vi "Test Zental PC  from Config file.vi"() -> ()   [LabVIEW 2009]
uses:
  LV-BME Interface/ChnlSettings.ctl
  DG Classes/BME_DG_Base/BME_DG_Base.lvclass
  DG Classes/BME_DG_Chnl/BME_DG_Chnl.lvclass
  DG Classes/BME_DG_System/BME_DG_System.lvclass
  POLARIS BME DG.lvlib
panel:
  out "error out 2":errorcluster
  in  "pathCalFiles":path=path "C:/CS Framework/LVSCC/LV2009/GPL/Projects/cs-framework/CSClass/CSPOLARIS/POLARIS BME DG"
  in  "pathParameterFile":path=path "C:/CS Framework/LVSCC/LV2009/GPL/Projects/cs-framework/CSClass/CSPOLARIS/POLARIS BME DG/test config  file.xml"
  out "stop error":errorcluster
  out "Problem Chnls out":string[](array[string])
  out "DelayFormulas":string[](array[string])=[" 10000.0095", "Delay Offset +0.819", "Pulspicker On + 0.013"]
  in  "Reset Error":bool
  out "error out":errorcluster
  in  "Update Delay formula":bool=TRUE
  in  "DelayFormula":string=" 10000.0095"
  in  "Aknowledge interrupts":bool=TRUE
  in  "stop 3":bool=TRUE
  in  "SetDelay":bool=TRUE
  in  "UpdateChnl":bool=TRUE
  in  "ChnlParameter":T2 {"ChnParam2write"."Delay (µs)" min=0.0 max=100000000.0 format="%.5f"}
  out "CountsRemains":i32=2147483647
  out "TriggerCounters":i32[](array[numeric])=[281, 0, 0, 0, -533591008, 0, 0, 0, 0]
  out "Interrupts":u32[](array[numeric])=[11153, 10240, 10240, 10240, 11008, 11008, 10240, 10240, 10240] format="%b"
  out "RemainingTriggers":T3(array[cluster])=[[{"Time Stamp"=timestamp(3421911180.6875 s since 1904-01-01), "Numeric"=1}, {"Time Stamp"=timestamp(3421911180.6875 s since 1904-01-01), "Numeric"=1}, {"Time Stamp"=timestamp(3421911180.6875 s since 1904-01-01), "Numeric"=1}, {"Time Stamp"=timestamp(3421911180.6875 s since 1904-01-01), "Numeric"=1}, {"Time Stamp"=timestamp(3421911180.6875 s since 1904-01-01), "Numeric"=9}, {"Time Stamp"=timestamp(3421911180.6875 s since 1904-01-01), "Numeric"=1}, {"Time Stamp"=timestamp(3421911180.6875 s since 1904-01-01), "Numeric"=1}, {"Time Stamp"=timestamp(3421911180.6875 s since 1904-01-01), "Numeric"=1}, {"Time Stamp"=timestamp(3421911180.6875 s since 1904-01-01), "Numeric"=1}], [{"Time Stamp"=timestamp(3421911180.6875 s since 1904-01-01), "Numeric"=10}, {"Time Stamp"=timestamp(3421911180.6875 s since 1904-01-01), "Numeric"=1}, {"Time Stamp"=timestamp(3421911180.6875 s since 1904-01-01), "Numeric"=1}, {"Time Stamp"=timestamp(3421911180.6875 s since 1904-01-01), "Numeric"=1}, {"Time Stamp"=timestamp(3421911180.6875 s since 1904-01-01), "Numeric"=9}, {"Time Stamp"=timestamp(3421911180.6875 s since 1904-01-01), "Numeric"=1}, {"Time Stamp"=timestamp(3421911180.6875 s since 1904-01-01), "Numeric"=1}, {"Time Stamp"=timestamp(3421911180.6875 s since 1904-01-01), "Numeric"=1}, {"Time Stamp"=timestamp(3421911180.6875 s since 1904-01-01), "Numeric"=1}], [{"Time Stamp"=timestamp(3421911180.6875 s since 1904-01-01), "Numeric"=10}, {"Time Stamp"=timestamp(3421911180.6875 s since 1904-01-01), "Numeric"=1}, {"Time Stamp"=timestamp(3421911180.6875 s since 1904-01-01), "Numeric"=1}, {"Time Stamp"=timestamp(3421911180.6875 s since 1904-01-01), "Numeric"=1}, {"Time Stamp"=timestamp(3421911180.6875 s since 1904-01-01), "Numeric"=609}, {"Time Stamp"=timestamp(3421911180.6875 s since 1904-01-01), "Numeric"=1}, {"Time Stamp"=timestamp(3421911180.6875 s since 1904-01-01), "Numeric"=1}, {"Time Stamp"=timestamp(3421911180.6875 s since 1904-01-01), "Numeric"=1}, {"Time Stamp"=timestamp(3421911180.6875 s since 1904-01-01), "Numeric"=1}]] {"Time Stamp" format="%<%I:%M:%S%3u %p>T"}
  in  "stop 2":bool=TRUE
  in  "ReadStatus":bool=TRUE
  in  "Activate":bool=TRUE
  in  "ResetModuloCounters":bool=TRUE
  in  "TriggerModulo":u32=4
  out "Modulo Settings":u32[](array[numeric])=[1, 10, 10]
  out "Chnls":T1[](array[typedef])=[{" Delay (µs)"=10000.0095, "On?"=TRUE, "PositiveVoltage?"=TRUE, "50OhmTerminated? "=TRUE, "25OhmOutput?"=FALSE}, {" Delay (µs)"=10000.829, "On?"=TRUE, "PositiveVoltage?"=TRUE, "50OhmTerminated? "=TRUE, "25OhmOutput?"=FALSE}, {" Delay (µs)"=10000.843, "On?"=TRUE, "PositiveVoltage?"=TRUE, "50OhmTerminated? "=TRUE, "25OhmOutput?"=FALSE}] {"Delay (µs)" min=0.0 max=100000000.0 format="%.5f"}
  in  "Selected Chnl":u16(ring)
  in  "Selected Card":u16(ring) items=["Master", "Servant"]
  in  "STOP":bool
  in  "ChnParam2write":T1={" Delay (µs)"=0.0, "On?"=TRUE, "PositiveVoltage?"=TRUE, "50OhmTerminated? "=TRUE, "25OhmOutput?"=FALSE} {"Delay (µs)" min=0.0 max=100000000.0 format="%.5f"}
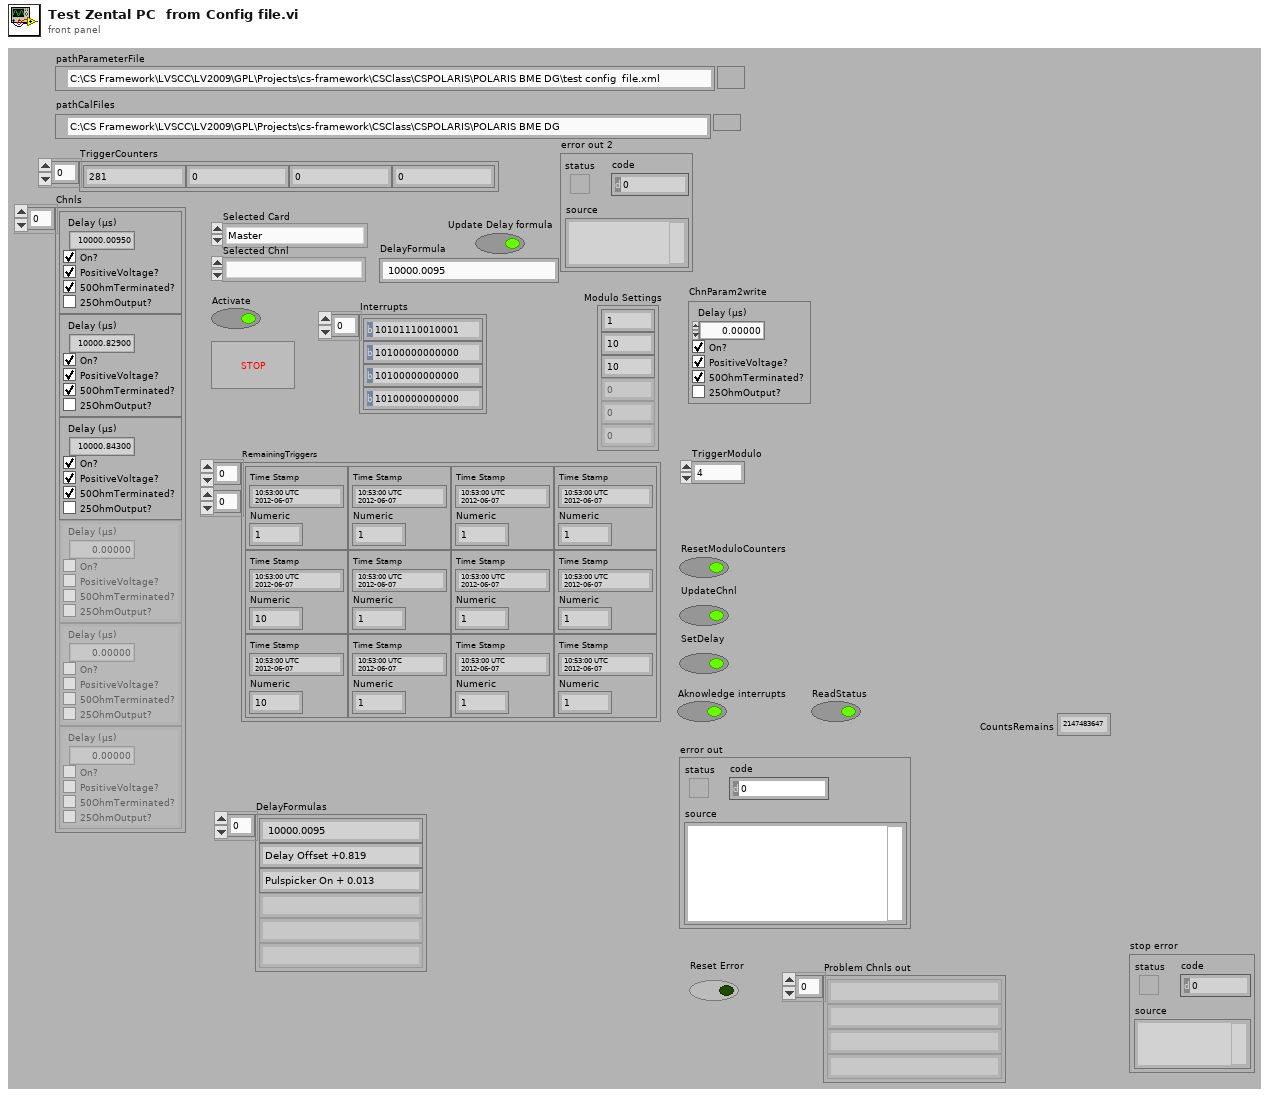
[diagram p1: front panel]
types:
  T1 = typedef "POLARIS BME DG.lvlib/ChnlSettings.ctl" = cluster{" Delay (µs)":dbl, "On?":bool, "PositiveVoltage?":bool, "50OhmTerminated? ":bool, "25OhmOutput?":bool}
  T2 = cluster{"ChnlName":string, "ChnParam2write":T1, "TriggerModulo":u32}
  T3 = cluster{"Time Stamp":timestamp, "Numeric":i32}[][]
  T4 = enum8{"Enabled", "Disabled", "Disabled and Grayed Out"}
  T5 = typedef "POLARIS BME DG.lvlib/BME_DG_TriggerSettings.ctl" = cluster{"Clock Source":T6, " clock modulo":u32, "TriggerEnabled?":bool, "trigger modulo ":i32, "InputTerminated?":bool, "Inhibit(µs)":dbl, "TriggerLevel":dbl, "PresetValue":i32, "InternalTrigger?":bool, "InternalArm?":bool, "SWTrigger?":bool, "RisingEdge?":bool, "StopOnPreset?":bool, "ResetWhenDone?":bool, "Gate Divider":i32, "PositiveGate?":bool}
  T6 = typedef "POLARIS BME DG.lvlib/ClockSource.ctl" = i32
  T7 = cluster{"ChnlName":string, "ChnParam2write":T1, "TriggerModulo":u32}[]
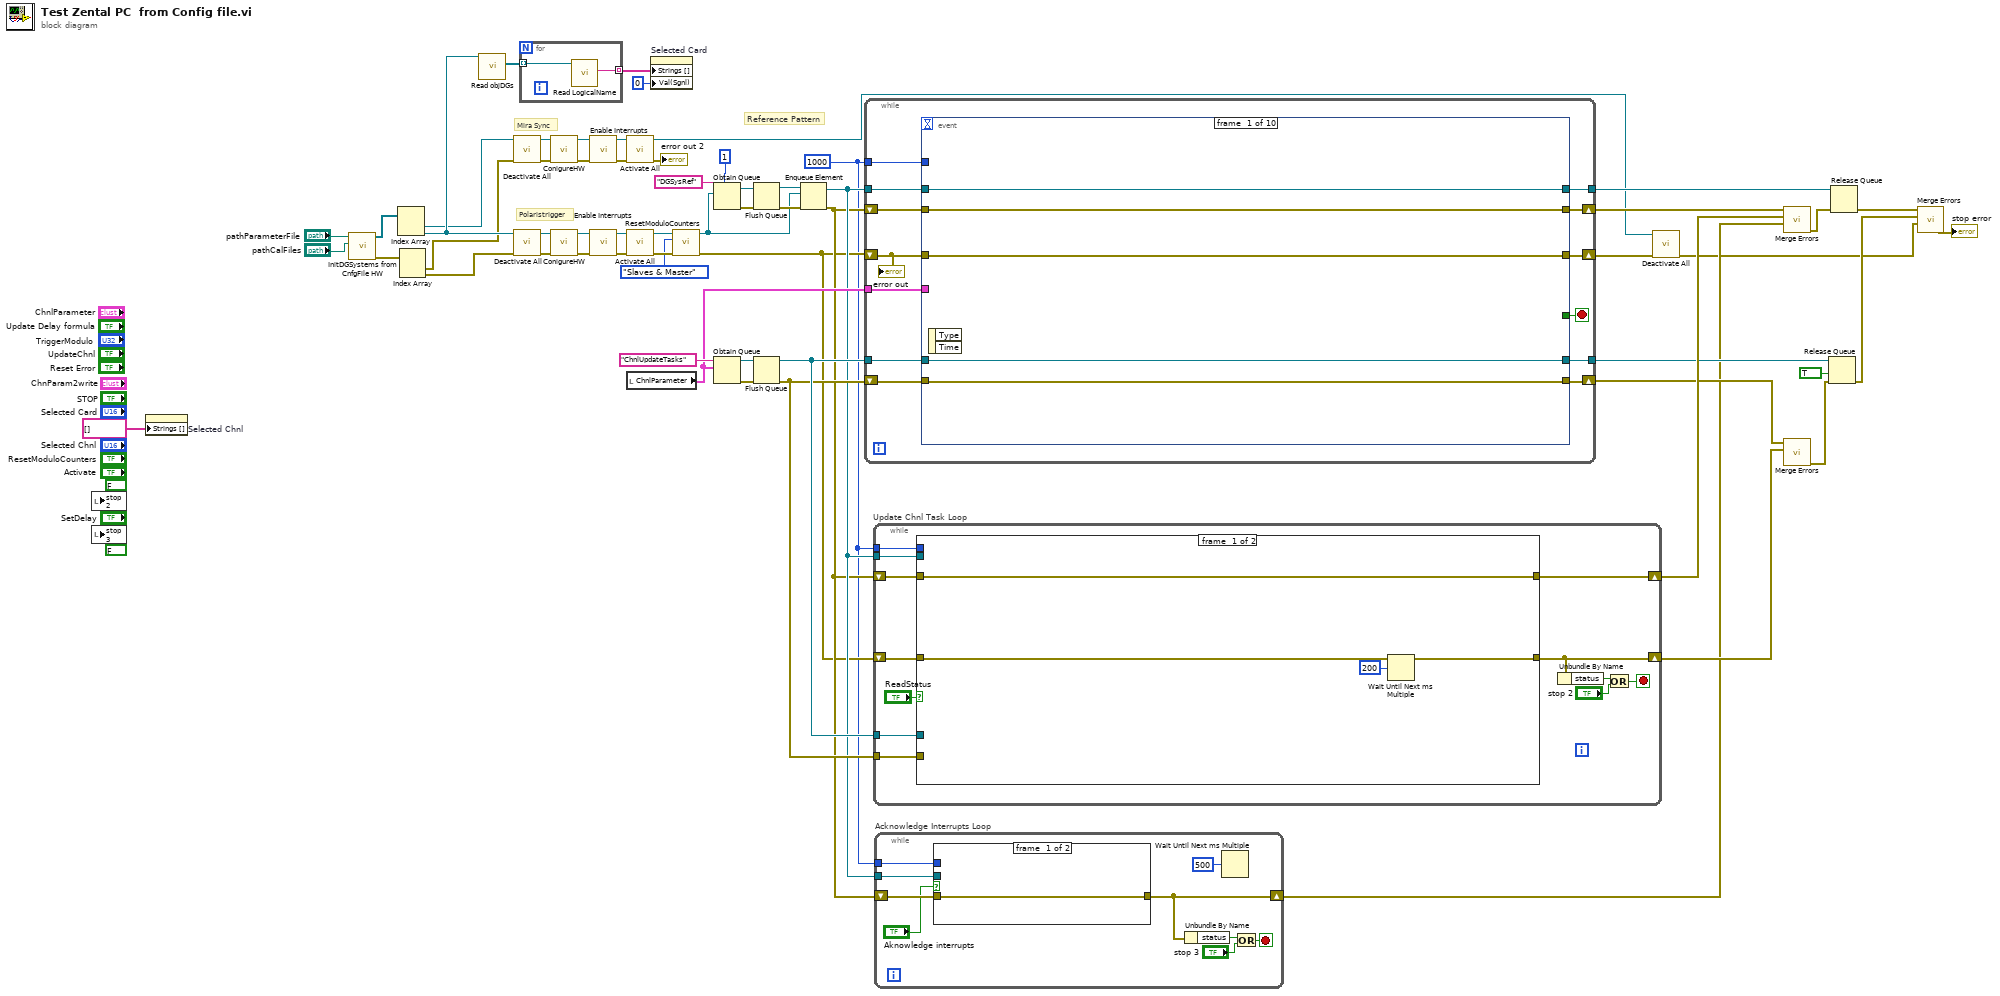
[diagram p0: block diagram]
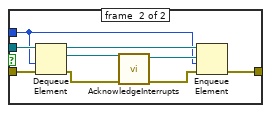
[diagram p2: hidden frame]
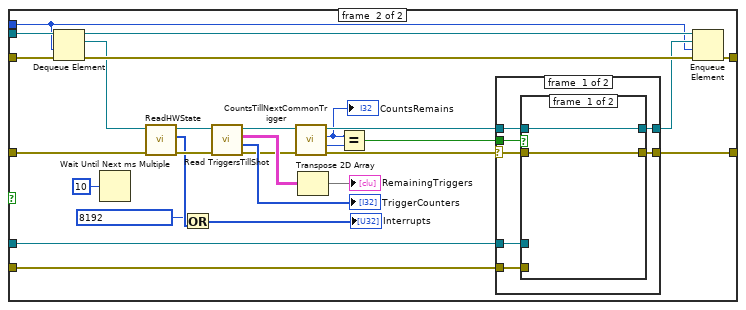
[diagram p3: hidden frame]
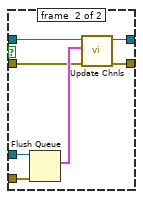
[diagram p4: hidden frame]
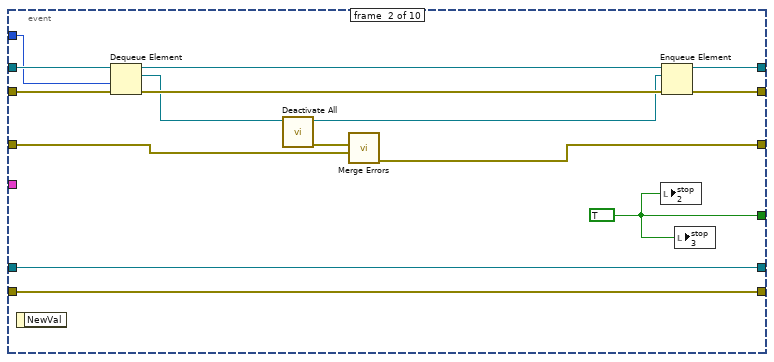
[diagram p6: hidden frame]
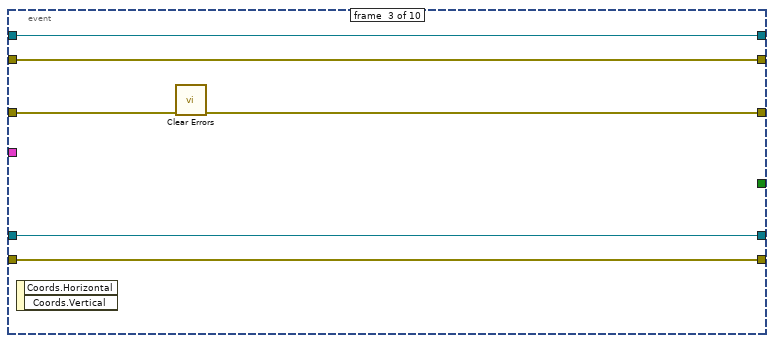
[diagram p7: hidden frame]
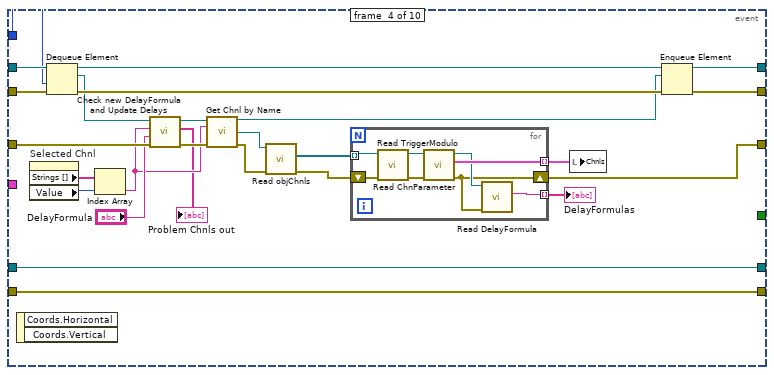
[diagram p8: hidden frame]
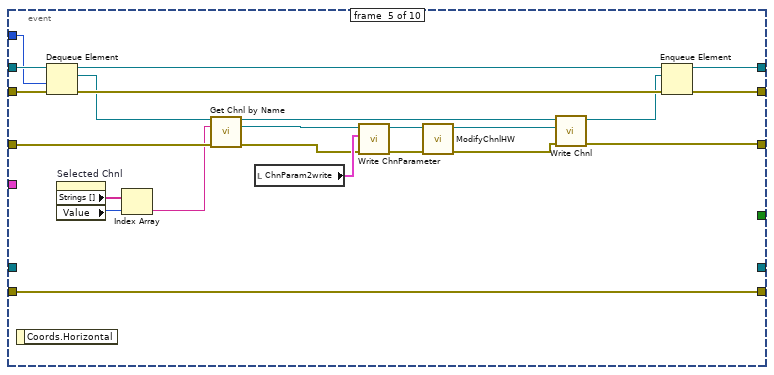
[diagram p9: hidden frame]
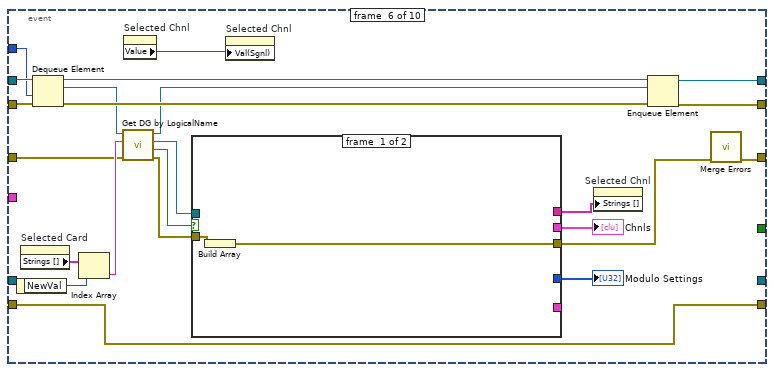
[diagram p10: hidden frame]
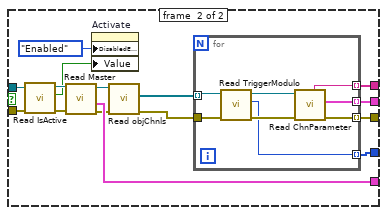
[diagram p11: hidden frame]
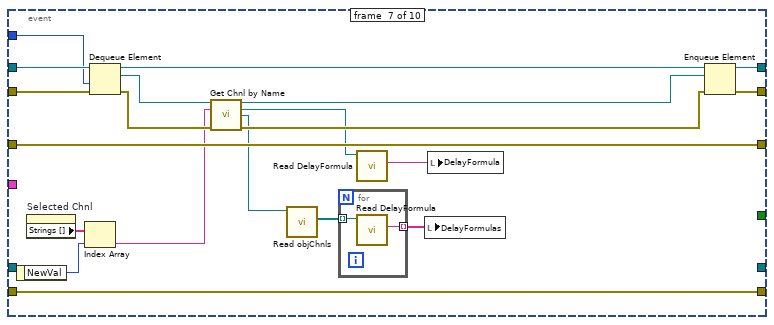
[diagram p12: hidden frame]
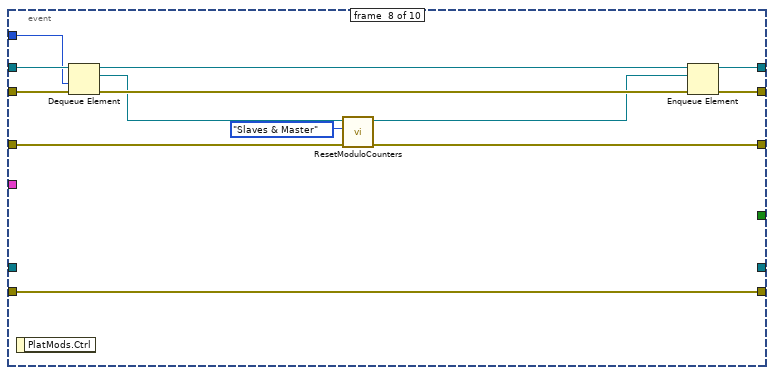
[diagram p13: hidden frame]
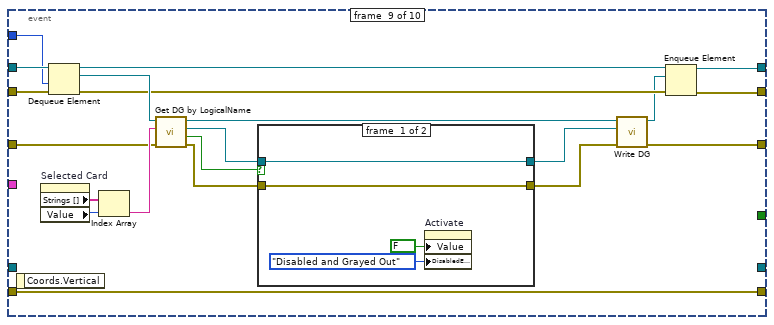
[diagram p14: hidden frame]
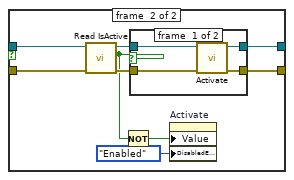
[diagram p15: hidden frame]
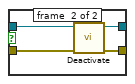
[diagram p16: hidden frame]
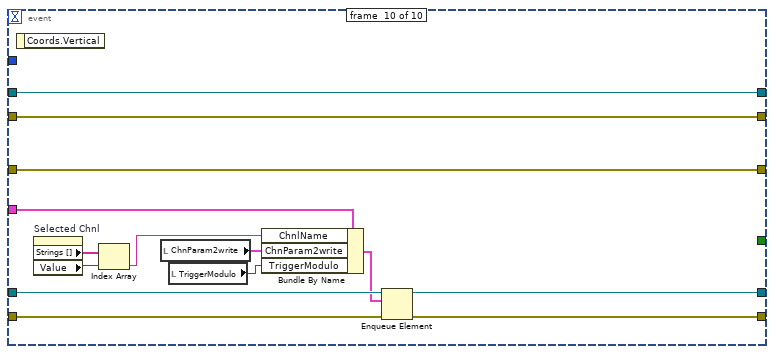
[diagram p17: hidden frame]
diagram:
  w21 = 1000 ("timeout in ms (-1)")
  # "Polaristrigger"
  # "Mira Sync"
  # "Reference Pattern"
  n1 = local write "stop 2"(FALSE ("stop 2")) -> ()
  n2 = local write "stop 3"(FALSE ("stop 3")) -> ()
  n3 = property on="Selected Chnl" class="Ring (strict)"("Strings []"=string[] []) -> ()  [unwired: 2 in, 2 out]
  n4 = call "InitDGSystems from CnfgFile HW.vi"("pathCalibrConsts"="pathCalFiles", "Config File"="pathParameterFile") -> ("Errors"=w7:errorcluster[], "DG Systems"=w16:refnum<class "BME_DG_System.lvclass">[])  [unwired: 8 in]
  n5 = Index Array(array=w16) -> (element #1=w8:refnum<class "BME_DG_System.lvclass">, element #2=w15:refnum<class "BME_DG_System.lvclass">)  [unwired: 2 in]
  n6 = Index Array(array=w7) -> (element #1=w5:errorcluster, element #2=w6:errorcluster)  [unwired: 2 in]
  n7 = call "Read objDGs.vi"("BME_DG_System in"=w15) -> ("objDGs"=w20:refnum<class "BME_DG_Base.lvclass">[])  [unwired: 8 in, 2 out]
  n8 = call "Deactivate All.vi"("error in (no error)"=w5, "BME_DG_System in"=w8) -> ("error out"=w10:errorcluster, "BME_DG_System out"=w9:refnum<class "BME_DG_System.lvclass">)  [unwired: 8 in]
  n9 = call "Deactivate All.vi"("error in (no error)"=w6, "BME_DG_System in"=w15) -> ("error out"=w38:errorcluster, "BME_DG_System out"=w39:refnum<class "BME_DG_System.lvclass">)  [unwired: 8 in]
  n10 = for {
    tunnel: w20 -> [w65] mode=indexing
    tunnel: [w64] -> w19 mode=indexing
    n11 = call "Read LogicalName.vi"("BME_DG_Base in"=w65) -> ("LogicalName"=w64:string)  [unwired: 8 in, 2 out]
  }
  n12 = call "ConigureHW.vi"("error in (no error)"=w10, "BME_DG_System in"=w9) -> ("error out"=w12:errorcluster, "BME_DG_System out"=w11:refnum<class "BME_DG_System.lvclass">)  [unwired: 8 in]
  n13 = call "ConigureHW.vi"("error in (no error)"=w38, "BME_DG_System in"=w39) -> ("error out"=w36:errorcluster, "BME_DG_System out"=w37:refnum<class "BME_DG_System.lvclass">)  [unwired: 8 in]
  n14 = call "Enable Interrupts.vi"("error in (no error)"=w12, "BME_DG_System in"=w11) -> ("error out"=w14:errorcluster, "BME_DG_System out"=w13:refnum<class "BME_DG_System.lvclass">)  [unwired: 8 in]
  n15 = call "Enable Interrupts.vi"("error in (no error)"=w36, "BME_DG_System in"=w37) -> ("error out"=w30:errorcluster, "BME_DG_System out"=w31:refnum<class "BME_DG_System.lvclass">)  [unwired: 8 in]
  n16 = call "Activate All.vi"("error in (no error)"=w14, "BME_DG_System in"=w13) -> ("error out"=→"error out 2":errorcluster, "BME_DG_System out"=w2:refnum<class "BME_DG_System.lvclass">)  [unwired: 8 in]
  n17 = call "Activate All.vi"("error in (no error)"=w30, "BME_DG_System in"=w31) -> ("error out"=w27:errorcluster, "BME_DG_System out"=w29:refnum<class "BME_DG_System.lvclass">)  [unwired: 8 in]
  n18 = local read "ChnlParameter"() -> (w47:T2)
  n19 = property on="Selected Card" class="Ring (strict)"("Strings []"=w19, "Val(Sgnl)"=u16 0 ("Value (Signaling)")) -> ()  [unwired: 2 in, 2 out]
  n20 = call "ResetModuloCounters.vi"("error in (no error)"=w27, "Enum"=enum16{"Slaves only", "Slaves & Master"}."Slaves & Master", "BME_DG_System in"=w29) -> ("error out"=w26:errorcluster, "BME_DG_System out"=w28:refnum<class "BME_DG_System.lvclass">)  [unwired: 7 in]
  n21 = Obtain Queue(max queue size (-1, unlimited)=1, name (unnamed)="DGSysRef", element data type=w28) -> (queue out=w55:refnum<queue>, error out=w53:errorcluster)  [unwired: 2 in, 1 out]
  n22 = Obtain Queue(name (unnamed)="ChnlUpdateTasks", element data type=w47) -> (queue out=w48:refnum<queue>, error out=w49:errorcluster)  [unwired: 3 in, 1 out]
  n23 = Flush Queue(queue=w55, error in (no error)=w53) -> (queue out=w54:refnum<queue>, error out=w52:errorcluster)  [unwired: 1 out]
  n24 = Flush Queue(queue=w48, error in (no error)=w49) -> (queue out=w44:refnum<queue>, error out=w43:errorcluster)  [unwired: 1 out]
  n25 = Enqueue Element(queue=w54, element=w28, error in (no error)=w52) -> (queue out=w35:refnum<queue>, error out=w34:errorcluster)  [unwired: 1 in, 1 out]
  n26 = while {
    shift-right: [w74] -> w4
    shift-left: w26 -> [w76]
    shift-right: [w72] -> w58
    shift-left: w34 -> [w73]
    tunnel: w35 -> [w77]
    tunnel: [w75] -> w60
    tunnel: w44 -> [w71]
    tunnel: w47 -> [w70]
    tunnel: [w68] -> w46
    shift-right: [w67] -> w42
    shift-left: w43 -> [w69]
    tunnel: w21 -> [w66]
    stop <- w78 stop-if-true
    n27 = event shown="[5] \"Selected Card\": Value Change" {
      selector: _ -> [_ _ _ _ _ _ _ _ _ _]
      dyn-events: _ -> [_ _ _ _ _ _ _ _ _ _]
      timeout: _ -> [_ _ _ _ _ _ _ _ _ _]
      tunnel: [_ w87 _ _ _ _ _ _ _ _] -> w78
      tunnel: w77 -> [w83 w96 w103 w129 w160 w173 w224 w244 w254 w300]
      tunnel: w76 -> [w82 w85 w104 w121 w151 w181 w229 w234 w262 w299]
      tunnel: [w83 w92 w103 w125 w156 w171 w222 w239 w248 w300] -> w75
      tunnel: [w82 w86 w99 w109 w140 w166 w229 w235 w255 w299] -> w74
      tunnel: w73 -> [w81 w95 w102 w128 w159 w172 w223 w242 w253 w296]
      tunnel: [w81 w93 w102 w126 w157 w170 w221 w240 w247 w296] -> w72
      tunnel: w71 -> [w80 w89 w101 w124 _ _ _ _ _ w291]
      tunnel: w70 -> [_ _ _ _ _ _ _ _ _ w295]
      tunnel: w69 -> [w79 w88 w100 w123 w155 w164 w228 w238 w246 w289]
      tunnel: [w80 w89 w101 w124 _ _ _ _ _ w288] -> w68
      tunnel: [w79 w88 w100 w123 w155 w164 w228 w238 w246 w287] -> w67
      tunnel: w66 -> [_ w84 _ w105 w139 w162 w210 w232 w245 _]
      event #0 {
        n28 = event-data() -> ()  [unwired: 1 in, 2 out]
      }
      event #1 {
        w87 = TRUE
        n29 = event-data() -> ()  [unwired: 1 in, 1 out]
        n30 = Dequeue Element(queue=w96, timeout in ms (-1)=w84, error in (no error)=w95) -> (queue out=w97:refnum<queue>, element=w90:refnum<class "BME_DG_System.lvclass">, error out=w94:errorcluster)  [unwired: 1 out]
        n31 = call "Deactivate All.vi"("BME_DG_System in"=w90) -> ("error out"=w98:errorcluster, "BME_DG_System out"=w91:refnum<class "BME_DG_System.lvclass">)  [unwired: 9 in]
        n32 = call <vilib>:"Merge Errors.vi"("error in 3 (no error)"=w85, "error in 2 (no error)"=w98) -> ("error out"=w86:errorcluster)  [unwired: 5 in]
        n33 = local write "stop 2"(w87) -> ()
        n34 = Enqueue Element(queue=w97, element=w91, error in (no error)=w94) -> (queue out=w92:refnum<queue>, error out=w93:errorcluster)  [unwired: 1 in, 1 out]
        n35 = local write "stop 3"(w87) -> ()
      }
      event #2 {
        n36 = event-data() -> ()  [unwired: 1 in, 2 out]
        n37 = call <vilib>:"Clear Errors.vi"("error in (no error)"=w104) -> ("error out"=w99:errorcluster)  [unwired: 6 in]
      }
      event #3 {
        n38 = event-data() -> ()  [unwired: 1 in, 2 out]
        n39 = property on="Selected Chnl" class="Ring (strict)"() -> ("Strings []"=w119:string[], "Value"=w120:u16)  [unwired: 2 in, 2 out]
        n40 = Dequeue Element(queue=w129, timeout in ms (-1)=w105, error in (no error)=w128) -> (queue out=w130:refnum<queue>, element=w122:refnum<class "BME_DG_System.lvclass">, error out=w127:errorcluster)  [unwired: 1 out]
        n41 = Index Array(array=w119, index=w120) -> (element=w108:string)
        n42 = call "Check new DelayFormula and Update Delays.vi"("error in (no error)"=w121, "Delay Formula"="DelayFormula", "ChnlName"=w108, "BME_DG_System in"=w122) -> ("error out"=w111:errorcluster, "Problem Chnls out"=→"Problem Chnls out":string[], "BME_DG_System out"=w113:refnum<class "BME_DG_System.lvclass">)  [unwired: 5 in]
        n43 = call "Get Chnl by Name.vi"("BME_DG_System in"=w113, "Chnl Name"=w108, "error in (no error)"=w111) -> ("BME_DG_System out"=w112:refnum<class "BME_DG_System.lvclass">, "Owner DG"=w114:refnum<class "BME_DG_Base.lvclass">, "error out"=w110:errorcluster)  [unwired: 7 in, 3 out]
        n44 = call-dynamic "Read objChnls.vi"("error in (no error)"=w110, "BME_DG_Base in"=w114) -> ("error out"=w115:errorcluster, "objChnls"=w117:refnum<class "BME_DG_Chnl.lvclass">[])  [unwired: 6 in, 2 out]
        n45 = for {
          tunnel: w117 -> [w137] mode=indexing
          tunnel: [w138] -> w116 mode=indexing
          shift-right: [w132] -> w109
          shift-left: w115 -> [w135]
          tunnel: [w131] -> w107 mode=indexing
          n46 = call-dynamic "Read TriggerModulo.vi"("error in (no error)"=w135, "BME_DG_Chnl in"=w137) -> ("error out"=w134:errorcluster, "BME_DG_Chnl out"=w136:refnum<class "BME_DG_Chnl.lvclass">)  [unwired: 7 in, 1 out]
          n47 = call-dynamic "Read ChnParameter.vi"("error in (no error)"=w134, "BME_DG_Chnl in"=w136) -> ("error out"=w132:errorcluster, "ChnParemater"=w138:T1, "BME_DG_Chnl out"=w133:refnum<class "BME_DG_Chnl.lvclass">)  [unwired: 4 in, 3 out]
          n48 = call-dynamic "Read DelayFormula.vi"("error in (no error)"=w132, "BME_DG_Chnl in"=w133) -> ("DelayFormula"=w131:string)  [unwired: 7 in, 2 out]
        }
        "DelayFormulas" <- w107
        n49 = local write "Chnls"(w116) -> ()
        n50 = Enqueue Element(queue=w130, element=w112, error in (no error)=w127) -> (queue out=w125:refnum<queue>, error out=w126:errorcluster)  [unwired: 1 in, 1 out]
      }
      event #4 {
        n51 = event-data() -> ()  [unwired: 1 in, 1 out]
        n52 = Dequeue Element(queue=w160, timeout in ms (-1)=w139, error in (no error)=w159) -> (queue out=w161:refnum<queue>, element=w152:refnum<class "BME_DG_System.lvclass">, error out=w158:errorcluster)  [unwired: 1 out]
        n53 = property on="Selected Chnl" class="Ring (strict)"() -> ("Strings []"=w153:string[], "Value"=w154:u16)  [unwired: 2 in, 2 out]
        n54 = Index Array(array=w153, index=w154) -> (element=w150:string)
        n55 = call "Get Chnl by Name.vi"("BME_DG_System in"=w152, "Chnl Name"=w150, "error in (no error)"=w151) -> ("BME_DG_System out"=w146:refnum<class "BME_DG_System.lvclass">, "BME_DG_Chnl"=w149:refnum<class "BME_DG_Chnl.lvclass">, "error out"=w147:errorcluster)  [unwired: 7 in, 3 out]
        n56 = local read "ChnParam2write"() -> (w148:T1)
        n57 = call-dynamic "Write ChnParameter.vi"("error in (no error)"=w147, "ChnParemater"=w148, "BME_DG_Chnl in"=w149) -> ("error out"=w143:errorcluster, "BME_DG_Chnl out"=w144:refnum<class "BME_DG_Chnl.lvclass">)  [unwired: 7 in]
        n58 = call-dynamic "ModifyChnlHW.vi"("error in (no error)"=w143, "BME_DG_Chnl in"=w144) -> ("error out"=w141:errorcluster, "BME_DG_Chnl out"=w142:refnum<class "BME_DG_Chnl.lvclass">)  [unwired: 8 in]
        n59 = call "Write Chnl.vi"("error in (no error)"=w141, "BME_DG_Chnl.lvclass"=w142, "BME_DG_System in"=w146) -> ("error out"=w140:errorcluster, "BME_DG_System out"=w145:refnum<class "BME_DG_System.lvclass">)  [unwired: 7 in]
        n60 = Enqueue Element(queue=w161, element=w145, error in (no error)=w158) -> (queue out=w156:refnum<queue>, error out=w157:errorcluster)  [unwired: 1 in, 1 out]
      }
      event #5 {
        n61 = event-data() -> ("NewVal"=w183:u16)  [unwired: 1 in]
        n62 = property on="Selected Card" class="Ring (strict)"() -> ("Strings []"=w184:string[])  [unwired: 2 in, 2 out]
        n63 = Dequeue Element(queue=w173, timeout in ms (-1)=w162, error in (no error)=w172) -> (queue out=w174:refnum<queue>, element=w169:refnum<class "BME_DG_System.lvclass">, error out=w175:errorcluster)  [unwired: 1 out]
        n64 = Index Array(array=w184, index=w183) -> (element=w182:string)
        n65 = call "Get DG by LogicalName.vi"("error in (no error)"=w181, "LogicalName"=w182, "BME_DG_System in"=w169) -> ("error out"=w167:errorcluster, "found?"=w180:bool, "BME_DG_Base.lvclass"=w179:refnum<class "BME_DG_Base.lvclass">, "BME_DG_System out"=w168:refnum<class "BME_DG_System.lvclass">)  [unwired: 5 in]
        n66 = property on="Selected Chnl" class="Ring (strict)"() -> ("Value"=w163:u16)  [unwired: 2 in, 2 out]
        n67 = case shown="False" w180 {
          tunnel: w179 -> [_ w194]
          tunnel: [_ w201] -> w178
          tunnel: [_ w200] -> w177
          tunnel: [_ w199] -> _
          tunnel: [_ w195] -> w176
          tunnel: w167 -> [w186 w191]
          tunnel: [w185 w189] -> w165
          frame #0 {
            n68 = Build Array(w186) -> (w185:errorcluster[])
          }
          frame #1 {
            n69 = call-dynamic "Read IsActive.vi"("error in (no error)"=w191, "BME_DG_Base in"=w194) -> ("error out"=w192:errorcluster, "Active?"=w187:bool, "BME_DG_Base out"=w193:refnum<class "BME_DG_Base.lvclass">)  [unwired: 7 in]
            n70 = call-dynamic "Read Master.vi"("error in (no error)"=w192, "BME_DG_Base in"=w193) -> ("error out"=w196:errorcluster, "TriggerSettings"=w199:T5, "BME_DG_Base out"=w197:refnum<class "BME_DG_Base.lvclass">)  [unwired: 6 in, 1 out]
            n71 = property on="Activate" class="Bool (strict)"("DisabledEnum"=T4."Enabled" ("Disabled"), "Value"=w187) -> ()  [unwired: 2 in, 2 out]
            n72 = call-dynamic "Read objChnls.vi"("error in (no error)"=w196, "BME_DG_Base in"=w197) -> ("error out"=w190:errorcluster, "objChnls"=w198:refnum<class "BME_DG_Chnl.lvclass">[])  [unwired: 6 in, 2 out]
            n73 = for {
              tunnel: w198 -> [w207] mode=indexing
              tunnel: [w209] -> w201 mode=indexing
              tunnel: [w208] -> w200 mode=indexing
              tunnel: [w202] -> w195 mode=indexing
              tunnel: w190 -> [w205]
              tunnel: [w203] -> w189 mode=indexing
              n74 = call-dynamic "Read TriggerModulo.vi"("error in (no error)"=w205, "BME_DG_Chnl in"=w207) -> ("error out"=w204:errorcluster, "TriggerModulo"=w202:i32, "BME_DG_Chnl out"=w206:refnum<class "BME_DG_Chnl.lvclass">)  [unwired: 7 in]
              n75 = call-dynamic "Read ChnParameter.vi"("error in (no error)"=w204, "BME_DG_Chnl in"=w206) -> ("error out"=w203:errorcluster, "ChnParemater"=w208:T1, "Name"=w209:string)  [unwired: 4 in, 3 out]
            }
          }
        }
        "Chnls" <- w177
        "Modulo Settings" <- w176
        n76 = property on="Selected Chnl" class="Ring (strict)"("Val(Sgnl)"=w163) -> ()  [unwired: 2 in, 2 out]
        n77 = property on="Selected Chnl" class="Ring (strict)"("Strings []"=w178) -> ()  [unwired: 2 in, 2 out]
        n78 = Enqueue Element(queue=w174, element=w168, error in (no error)=w175) -> (queue out=w171:refnum<queue>, error out=w170:errorcluster)  [unwired: 1 in, 1 out]
        n79 = call <vilib>:"Merge Errors.vi"("error array in"=w165) -> ("error out"=w166:errorcluster)  [unwired: 6 in]
      }
      event #6 {
        n80 = event-data() -> ("NewVal"=w226:u16)  [unwired: 1 in]
        n81 = property on="Selected Chnl" class="Ring (strict)"() -> ("Strings []"=w227:string[])  [unwired: 2 in, 2 out]
        n82 = Index Array(array=w227, index=w226) -> (element=w216:string)
        n83 = Dequeue Element(queue=w224, timeout in ms (-1)=w210, error in (no error)=w223) -> (queue out=w225:refnum<queue>, element=w217:refnum<class "BME_DG_System.lvclass">, error out=w219:errorcluster)  [unwired: 1 out]
        n84 = call "Get Chnl by Name.vi"("BME_DG_System in"=w217, "Chnl Name"=w216, "error in (no error)"=w219) -> ("BME_DG_System out"=w220:refnum<class "BME_DG_System.lvclass">, "BME_DG_Chnl"=w214:refnum<class "BME_DG_Chnl.lvclass">, "Owner DG"=w213:refnum<class "BME_DG_Base.lvclass">, "error out"=w218:errorcluster)  [unwired: 7 in, 2 out]
        n85 = call-dynamic "Read objChnls.vi"("BME_DG_Base in"=w213) -> ("objChnls"=w212:refnum<class "BME_DG_Chnl.lvclass">[])  [unwired: 7 in, 3 out]
        n86 = for {
          tunnel: w212 -> [w231] mode=indexing
          tunnel: [w230] -> w211 mode=indexing
          n87 = call-dynamic "Read DelayFormula.vi"("BME_DG_Chnl in"=w231) -> ("DelayFormula"=w230:string)  [unwired: 8 in, 2 out]
        }
        n88 = call-dynamic "Read DelayFormula.vi"("BME_DG_Chnl in"=w214) -> ("DelayFormula"=w215:string)  [unwired: 8 in, 2 out]
        n89 = local write "DelayFormulas"(w211) -> ()
        n90 = local write "DelayFormula"(w215) -> ()
        n91 = Enqueue Element(queue=w225, element=w220, error in (no error)=w218) -> (queue out=w222:refnum<queue>, error out=w221:errorcluster)  [unwired: 1 in, 1 out]
      }
      event #7 {
        n92 = event-data() -> ()  [unwired: 1 in, 1 out]
        n93 = Dequeue Element(queue=w244, timeout in ms (-1)=w232, error in (no error)=w242) -> (queue out=w243:refnum<queue>, element=w237:refnum<class "BME_DG_System.lvclass">, error out=w241:errorcluster)  [unwired: 1 out]
        n94 = call "ResetModuloCounters.vi"("error in (no error)"=w234, "Enum"=enum16{"Slaves only", "Slaves & Master"}."Slaves & Master", "BME_DG_System in"=w237) -> ("error out"=w235:errorcluster, "BME_DG_System out"=w236:refnum<class "BME_DG_System.lvclass">)  [unwired: 7 in]
        n95 = Enqueue Element(queue=w243, element=w236, error in (no error)=w241) -> (queue out=w239:refnum<queue>, error out=w240:errorcluster)  [unwired: 1 in, 1 out]
      }
      event #8 {
        n96 = event-data() -> ()  [unwired: 1 in, 1 out]
        n97 = property on="Selected Card" class="Ring (strict)"() -> ("Strings []"=w265:string[], "Value"=w264:u16)  [unwired: 2 in, 2 out]
        n98 = Dequeue Element(queue=w254, timeout in ms (-1)=w245, error in (no error)=w253) -> (queue out=w251:refnum<queue>, element=w252:refnum<class "BME_DG_System.lvclass">, error out=w250:errorcluster)  [unwired: 1 out]
        n99 = Index Array(array=w265, index=w264) -> (element=w263:string)
        n100 = call "Get DG by LogicalName.vi"("error in (no error)"=w262, "LogicalName"=w263, "BME_DG_System in"=w252) -> ("error out"=w260:errorcluster, "found?"=w256:bool, "BME_DG_Base.lvclass"=w261:refnum<class "BME_DG_Base.lvclass">, "BME_DG_System out"=w257:refnum<class "BME_DG_System.lvclass">)  [unwired: 5 in]
        n101 = case shown="True" w256 {
          tunnel: w261 -> [w269 w276]
          tunnel: w260 -> [w268 w274]
          tunnel: [w268 w278] -> w259
          tunnel: [w269 w277] -> w258
          frame #0 {
            n102 = property on="Activate" class="Bool (strict)"("Value"=FALSE ("Activate"), "DisabledEnum"=T4."Disabled and Grayed Out" ("Disabled")) -> ()  [unwired: 2 in, 2 out]
          }
          frame #1 {
            n103 = call-dynamic "Read IsActive.vi"("error in (no error)"=w274, "BME_DG_Base in"=w276) -> ("error out"=w273:errorcluster, "Active?"=w272:bool, "BME_DG_Base out"=w275:refnum<class "BME_DG_Base.lvclass">)  [unwired: 7 in]
            n104 = Not(x=w272) -> (.not. x?=w270:bool)
            n105 = case shown="True" w272 {
              tunnel: [w282 w284] -> w278
              tunnel: [w281 w285] -> w277
              tunnel: w275 -> [w280 w286]
              tunnel: w273 -> [w279 w283]
              frame #0 {
                n106 = call-dynamic "Activate.vi"("error in (no error)"=w279, "BME_DG_Base in"=w280) -> ("error out"=w282:errorcluster, "BME_DG_Base out"=w281:refnum<class "BME_DG_Base.lvclass">)  [unwired: 8 in]
              }
              frame #1 {
                n107 = call-dynamic "Deactivate.vi"("error in (no error)"=w283, "BME_DG_Base in"=w286) -> ("error out"=w284:errorcluster, "BME_DG_Base out"=w285:refnum<class "BME_DG_Base.lvclass">)  [unwired: 8 in]
              }
            }
            n108 = property on="Activate" class="Bool (strict)"("Value"=w270, "DisabledEnum"=T4."Enabled" ("Disabled")) -> ()  [unwired: 2 in, 2 out]
          }
        }
        n109 = call "Write DG.vi"("error in (no error)"=w259, "BME_DG_Base"=w258, "BME_DG_System in"=w257) -> ("error out"=w255:errorcluster, "BME_DG_System out"=w249:refnum<class "BME_DG_System.lvclass">)  [unwired: 7 in]
        n110 = Enqueue Element(queue=w251, element=w249, error in (no error)=w250) -> (queue out=w248:refnum<queue>, error out=w247:errorcluster)  [unwired: 1 in, 1 out]
      }
      event #9 {
        n111 = event-data() -> ()  [unwired: 1 in, 1 out]
        n112 = property on="Selected Chnl" class="Ring (strict)"() -> ("Strings []"=w297:string[], "Value"=w298:u16)  [unwired: 2 in, 2 out]
        n113 = Index Array(array=w297, index=w298) -> (element=w294:string)
        n114 = local read "ChnParam2write"() -> (w293:T1)
        n115 = local read "TriggerModulo"() -> (w292:u32)
        n116 = Bundle By Name(cluster=w295, "ChnlName"=w294, "ChnParam2write"=w293, "TriggerModulo"=w292) -> (w290:T2)
        n117 = Enqueue Element(queue=w291, element=w290, error in (no error)=w289) -> (queue out=w288:refnum<queue>, error out=w287:errorcluster)  [unwired: 1 in, 1 out]
      }
    }
    "error out" <- w76
  }
  n118 = while "Update Chnl Task Loop" {
    tunnel: w35 -> [w309]
    shift-right: [w307] -> w57
    shift-left: w34 -> [w308]
    shift-right: [w304] -> w41
    shift-left: w26 -> [w306]
    tunnel: w44 -> [w303]
    tunnel: w43 -> [w302]
    tunnel: w21 -> [w301]
    stop <- w311 stop-if-true
    n119 = case shown="True" "ReadStatus" {
      tunnel: w309 -> [_ w341]
      tunnel: w308 -> [w314 w340]
      tunnel: [w314 w339] -> w307
      tunnel: w306 -> [w313 w337]
      tunnel: [w313 w323] -> w304
      tunnel: w303 -> [_ w327]
      tunnel: w302 -> [_ w326]
      tunnel: w301 -> [_ w316]
      frame #0 {
        n120 = Wait Until Next ms Multiple(millisecond multiple=u32 200) -> ()  [unwired: 1 out]
      }
      frame #1 {
        n121 = Dequeue Element(queue=w341, timeout in ms (-1)=w316, error in (no error)=w340) -> (queue out=w342:refnum<queue>, element=w338:refnum<class "BME_DG_System.lvclass">, error out=w343:errorcluster)  [unwired: 1 out]
        n122 = Wait Until Next ms Multiple(millisecond multiple=u32 10) -> ()  [unwired: 1 out]
        n123 = call "ReadHWState.vi"("error in (no error)"=w337, "BME_DG_System in"=w338) -> ("error out"=w336:errorcluster, "Interrupts"=w332:u32[], "BME_DG_System out"=w335:refnum<class "BME_DG_System.lvclass">)  [unwired: 7 in]
        n124 = Or(x=u32 8192, y=w332) -> (x .or. y?=→"Interrupts":u32[])
        n125 = call "Read TriggersTillShot.vi"("error in (no error)"=w336, "BME_DG_System in"=w335) -> ("error out"=w328:errorcluster, "TriggerCounters"=→"TriggerCounters":i32[], "RemainingTriggers"=w334:T3, "BME_DG_System out"=w329:refnum<class "BME_DG_System.lvclass">)  [unwired: 6 in]
        n126 = call "CountsTillNextCommonTrigger.vi"("error in (no error)"=w328, "BME_DG_System in"=w329) -> ("error out"=w325:errorcluster, "LeastCommonMult"=w320:i32, "CountsRemains"=w321:i32, "BME_DG_System out"=w324:refnum<class "BME_DG_System.lvclass">)  [unwired: 6 in]
        "CountsRemains" <- w321
        n127 = Transpose 2D Array(2D array=w334) -> (transposed array=→"RemainingTriggers":T3)
        n128 = Equal?(x=w321, y=w320) -> (x = y?=w319:bool)
        n129 = case shown="No Error" w325 {
          selector: w325 -> [w347 w360]
          tunnel: w327 -> [w350 _]
          tunnel: w326 -> [w349 _]
          tunnel: w324 -> [w348 w361]
          tunnel: [w346 w360] -> w323
          tunnel: [w345 w361] -> w322
          tunnel: w319 -> [w344 _]
          frame #0 {
            n130 = case shown="True" w344 {
              tunnel: w350 -> [_ w359]
              tunnel: w349 -> [_ w358]
              tunnel: w348 -> [w352 w357]
              tunnel: w347 -> [w351 w355]
              tunnel: [w351 w354] -> w346
              tunnel: [w352 w353] -> w345
              frame #0 {
              }
              frame #1 {
                n131 = Flush Queue(queue=w359, error in (no error)=w358) -> (remaining elements=w356:T7)  [unwired: 2 out]
                n132 = call "Update Chnls.vi"("error in (no error)"=w355, "ChnlSettings"=w356, "BME_DG_System in"=w357) -> ("error out"=w354:errorcluster, "BME_DG_System out"=w353:refnum<class "BME_DG_System.lvclass">)  [unwired: 7 in]
              }
            }
          }
          frame #1 {
          }
        }
        n133 = Enqueue Element(queue=w342, element=w322, timeout in ms (-1)=w316, error in (no error)=w343) -> (error out=w339:errorcluster)  [unwired: 2 out]
      }
    }
    n134 = Unbundle By Name(w304) -> ("status"=w310:bool)
    n135 = Or(x=w310, y="stop 2") -> (x .or. y?=w311:bool)
  }
  n136 = while "Acknowledge Interrupts Loop" {
    tunnel: w35 -> [w367]
    shift-right: [w365] -> w32
    shift-left: w34 -> [w366]
    tunnel: w21 -> [w362]
    stop <- w369 stop-if-true
    n137 = case shown="True" "Aknowledge interrupts" {
      tunnel: w367 -> [_ w380]
      tunnel: w366 -> [w371 w379]
      tunnel: [w371 w378] -> w365
      tunnel: w362 -> [_ w372]
      frame #0 {
      }
      frame #1 {
        n138 = Dequeue Element(queue=w380, timeout in ms (-1)=w372, error in (no error)=w379) -> (queue out=w377:refnum<queue>, element=w376:refnum<class "BME_DG_System.lvclass">, error out=w375:errorcluster)  [unwired: 1 out]
        n139 = call "AcknowledgeInterrupts.vi"("error in (no error)"=w375, "BME_DG_System in"=w376) -> ("error out"=w373:errorcluster, "BME_DG_System out"=w374:refnum<class "BME_DG_System.lvclass">)  [unwired: 8 in]
        n140 = Enqueue Element(queue=w377, element=w374, timeout in ms (-1)=w372, error in (no error)=w373) -> (error out=w378:errorcluster)  [unwired: 2 out]
      }
    }
    n141 = Unbundle By Name(w365) -> ("status"=w368:bool)
    n142 = Wait Until Next ms Multiple(millisecond multiple=u32 500) -> ()  [unwired: 1 out]
    n143 = Or(x=w368, y="stop 3") -> (x .or. y?=w369:bool)
  }
  n144 = call "Deactivate All.vi"("error in (no error)"=w4, "BME_DG_System in"=w2) -> ("error out"=w3:errorcluster)  [unwired: 8 in, 1 out]
  n145 = call <vilib>:"Merge Errors.vi"("error in 3 (no error)"=w32, "error in 2 (no error)"=w57, "error in 1 (no error)"=w58) -> ("error out"=w59:errorcluster)  [unwired: 4 in]
  n146 = call <vilib>:"Merge Errors.vi"("error in 2 (no error)"=w41, "error in 1 (no error)"=w42) -> ("error out"=w40:errorcluster)  [unwired: 5 in]
  n147 = Release Queue(queue=w46, force destroy? (F)=TRUE, error in (no error)=w40) -> (error out=w23:errorcluster)  [unwired: 2 out]
  n148 = Release Queue(queue=w60, error in (no error)=w59) -> (error out=w24:errorcluster)  [unwired: 1 in, 2 out]
  n149 = call <vilib>:"Merge Errors.vi"("error in 3 (no error)"=w3, "error in 2 (no error)"=w23, "error in 1 (no error)"=w24) -> ("error out"=→"stop error":errorcluster)  [unwired: 4 in]
